vi "Arcade Drive with Joysticks.vi"(10 "Y Axis":dbl, 11 "X Axis":dbl) -> (2 "Speed":dbl, 3 "Turn":dbl)   [LabVIEW 2016]
uses:
  <vilib>/Rock Robotics/Network Tables/NT Read Number.vi
  <vilib>/Rock Robotics/Network Tables/NT Read Boolean.vi
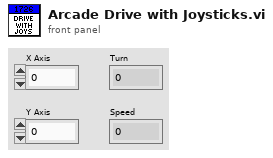
[diagram p1: front panel]
types:
  T1 = cluster{"Numeric":dbl, "Numeric":dbl, "Boolean":bool, "Numeric":dbl}
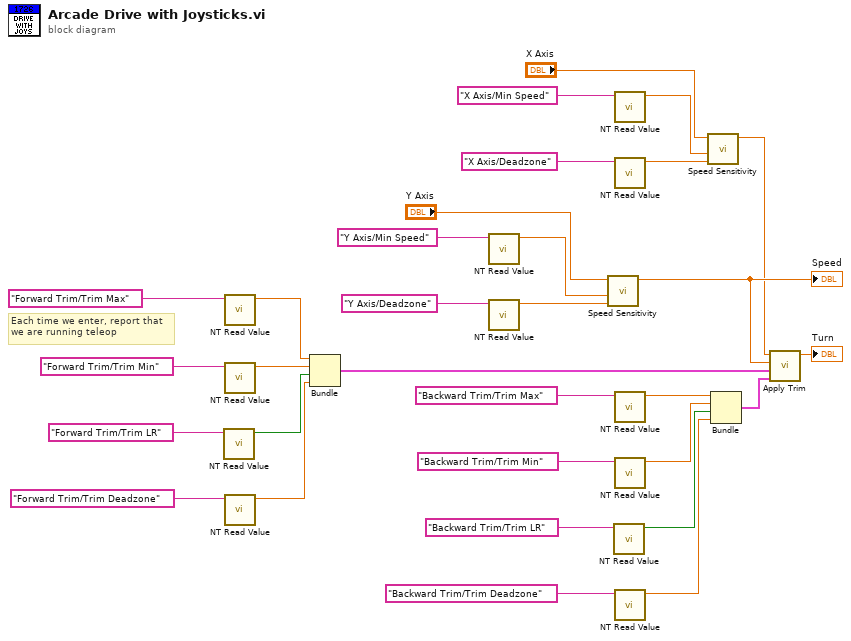
[diagram p0: block diagram]
diagram:
  # "Each time we enter, report that\nwe are running teleop"
  n1 = call-poly <vilib>:"NT Read Value.vi"("Name"="Forward Trim/Trim LR") -> ("Boolean"=w9:bool)  [unwired: 9 in, 1 out]
  n2 = call-poly <vilib>:"NT Read Value.vi"("Name"="Forward Trim/Trim Max") -> ("Numeric"=w7:dbl)  [unwired: 9 in, 1 out]
  n3 = call-poly <vilib>:"NT Read Value.vi"("Name"="Forward Trim/Trim Min") -> ("Numeric"=w8:dbl)  [unwired: 9 in, 1 out]
  n4 = call-poly <vilib>:"NT Read Value.vi"("Name"="Forward Trim/Trim Deadzone") -> ("Numeric"=w6:dbl)  [unwired: 9 in, 1 out]
  n5 = Bundle("Numeric"=w7, "Numeric"=w8, "Boolean"=w9, "Numeric"=w6) -> (w12:T1)  [unwired: 1 in]
  n6 = call-poly <vilib>:"NT Read Value.vi"("Name"="Y Axis/Min Speed") -> ("Numeric"=w29:dbl)  [unwired: 9 in, 1 out]
  n7 = call-poly <vilib>:"NT Read Value.vi"("Name"="Y Axis/Deadzone") -> ("Numeric"=w30:dbl)  [unwired: 9 in, 1 out]
  n8 = call "Speed Sensitivity.vi"("Deadzone"=w30, "Min Speed"=w29, "Input"="Y Axis") -> ("Output"=w31:dbl)  [unwired: 8 in]
  "Speed" <- w31
  n9 = call-poly <vilib>:"NT Read Value.vi"("Name"="Backward Trim/Trim LR") -> ("Boolean"=w20:bool)  [unwired: 9 in, 1 out]
  n10 = call-poly <vilib>:"NT Read Value.vi"("Name"="X Axis/Min Speed") -> ("Numeric"=w27:dbl)  [unwired: 9 in, 1 out]
  n11 = call-poly <vilib>:"NT Read Value.vi"("Name"="X Axis/Deadzone") -> ("Numeric"=w28:dbl)  [unwired: 9 in, 1 out]
  n12 = call-poly <vilib>:"NT Read Value.vi"("Name"="Backward Trim/Trim Max") -> ("Numeric"=w18:dbl)  [unwired: 9 in, 1 out]
  n13 = call-poly <vilib>:"NT Read Value.vi"("Name"="Backward Trim/Trim Min") -> ("Numeric"=w19:dbl)  [unwired: 9 in, 1 out]
  n14 = call-poly <vilib>:"NT Read Value.vi"("Name"="Backward Trim/Trim Deadzone") -> ("Numeric"=w17:dbl)  [unwired: 9 in, 1 out]
  n15 = call "Speed Sensitivity.vi"("Deadzone"=w28, "Min Speed"=w27, "Input"="X Axis") -> ("Output"=w11:dbl)  [unwired: 8 in]
  n16 = Bundle("Numeric"=w18, "Numeric"=w19, "Boolean"=w20, "Numeric"=w17) -> (w22:T1)  [unwired: 1 in]
  n17 = call "Apply Trim.vi"("Backwards Tuning"=w22, "Forward Tuning"=w12, "Speed"=w31, "Turn"=w11) -> ("Trimmed Turn"=→"Turn":dbl)  [unwired: 7 in]
